vi "Variant to JSON Text.vi"(4 "LVClass Serializer":refnum<class "JSONtext LVClass Serializer.lvclass">, 5 "enable LabVIEW extensions? (T)":bool=TRUE, 6 "Pretty Print?":bool, 8 "error in (no error)":errorcluster, 10 "Variant":variant) -> (0 "error out":errorcluster, 1 "Name of data in Variant":string, 3 "<JSON>":string)   [LabVIEW 2017, in "JSONtext.lvlib"]
doc: "Converts a LabVIEW datatype (<b>Variant</b>) into a JSON value. \n\nStrings or Arrays of strings marked with a leading \"<JSON>\" tag in their name (including inside clusters) are treated as already being valid JSON. Strings not marked as <JSON> are quoted and escaped as a JSON String. Note that JSONtext.lvlib functions that produce JSON have their outputs labelled \"<JSON>\", so that they may be used as inputs to other functions.\n\nTwo types of LabVIEW Clusters are supported: either with all named elements, which are converted to JSON Objects, or all unnamed elements (or elements just named \"<JSON>\"), which are converted to a JSON Array. Handling of mixed clusters with some named and some unnamed in undefined (currently, this VI will use the first element to determine whether to convert to an Object or Array)."
uses:
  JSONtext.lvlib
  LVClass Serializer/JSONtext LVClass Serializer.lvclass
  <vilib>/Utility/Data Type/Type Definitions/Data Type.ctl
  support/Remove trailing zeros.vi
  support/quote and escape json string 2.vi
  support/Format JSON Object.vi
  <vilib>/Utility/Data Type/NI_Data Type.lvlib
  <vilib>/JDP Science/JDP Science Common Utilities/JDP Utility.lvlib
  <vilib>/JDP Science/JDP Science Common Utilities/Timestamp/JDP Timestamp.lvlib
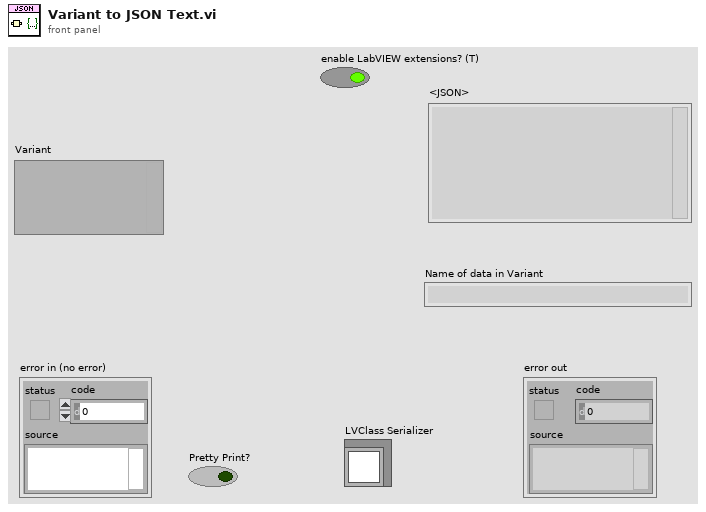
[diagram p1: front panel]
types:
  T1 = typedef "NI_Data Type.lvlib/Data Type.ctl" = enum8{"Invalid Type", "Void", "I8", "I16", "I32", "I64", "U8", "U16", "U32", "U64", "Single Float", "Double Float", "Extended Float", "Single Complex", "Double Complex", "Extended Complex", "Enum U8", "Enum U16", "Enum U32", "Enum U64", "Single Float With Unit", "Double Float With Unit", "Extended Float With Unit", "Single Complex with Unit", "Double Complex with Unit", "Extended Complex with Unit", "Boolean", "String", "Path", "Picture", "Tag", "Array", "Cluster", "Variant", "LV Variant", "Waveform", "Timestamp", "Digital Waveform", "Digital Data", "ExpressData", "Refnum", "External Data", "VI", "Poly VI", "LabVIEW Class Instance", "Fixed Point"}
  T2 = typedef "JSONtext.lvlib/Tag Type.ctl" = enum16{"No Tag", "<JSON>", "<JOBJ>"}
  T3 = cluster{"<JSON>attributes":string, "t0":timestamp, "dt":dbl, "Y":dbl[]}
  T4 = typedef "NI_Data Type.lvlib/Refnum Type.ctl" = enum16{"NotARefnum", "UnknownRefnum", "Generic", "Datalog", "ByteStream", "Device", "Occurence", "TCPNetConnection", "Auto", "Menu", "Imaq", "Hardware", "DataSocket", "Visa", "IVI", "UDPNetConnection", "Notifier", "Queue", "Irda", "EventReg", "DotNet", "UserEvent", "Callback", "UNUSED_EMPTY_POSITION", "BlueToothNetConnection", "LVObjApp", "LVObjVI", "LVObjUnknown", "GenericClass", "UserDefinedRefnumTag", "DataValue", "RT FIFO", "TDMS File"}
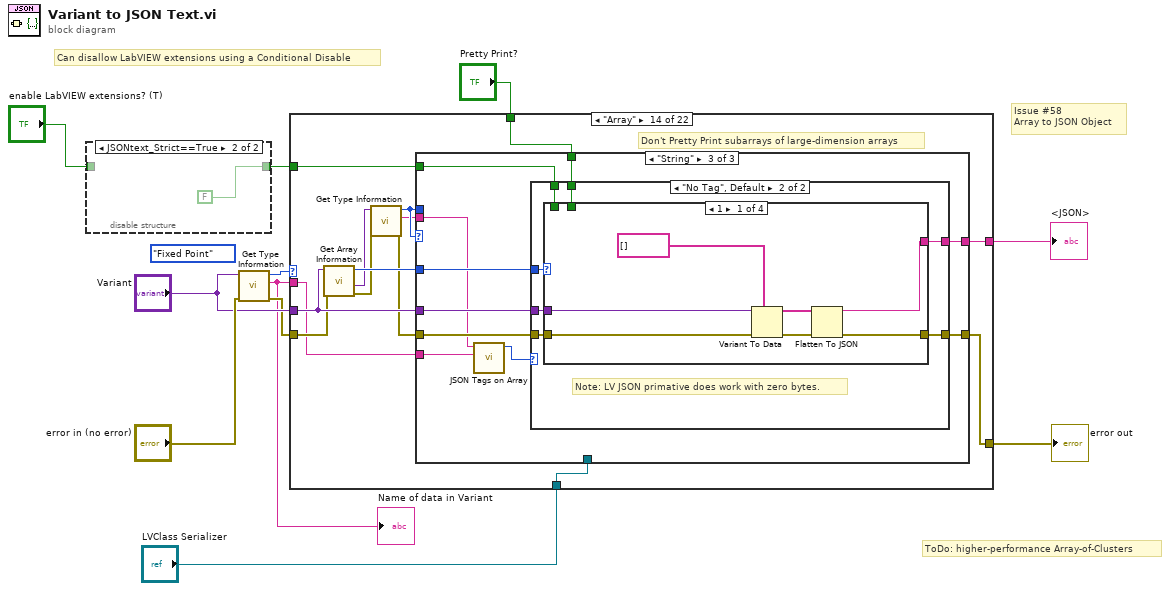
[diagram p0: block diagram]
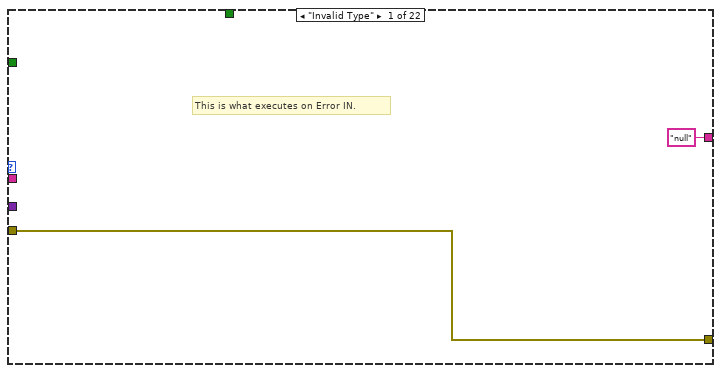
[diagram p3: hidden frame]
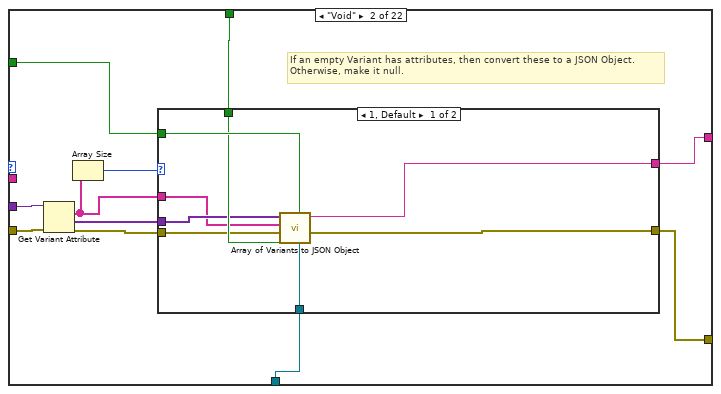
[diagram p4: hidden frame]
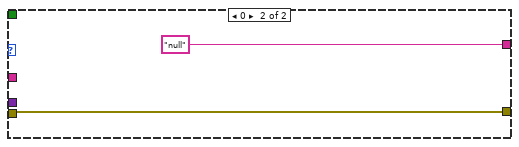
[diagram p5: hidden frame]
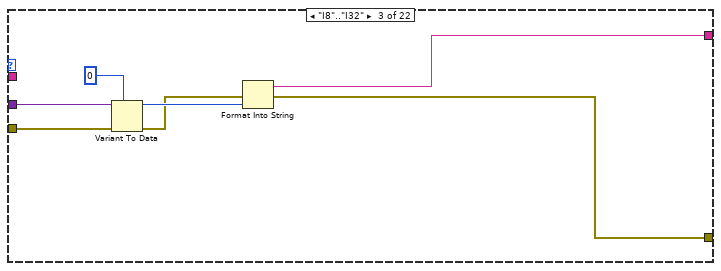
[diagram p6: hidden frame]
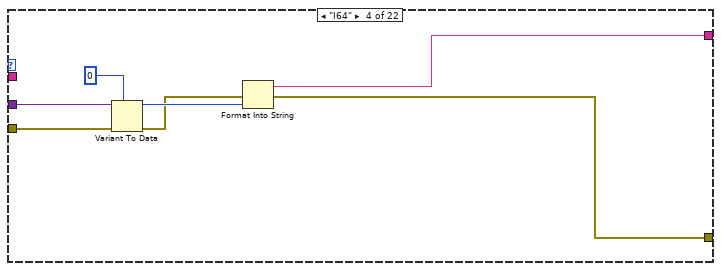
[diagram p7: hidden frame]
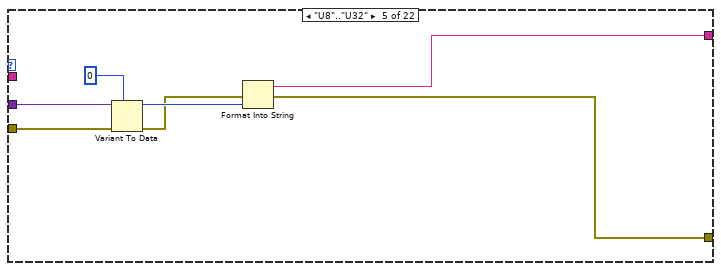
[diagram p8: hidden frame]
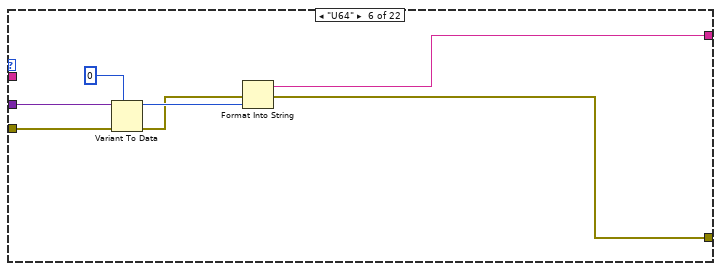
[diagram p9: hidden frame]
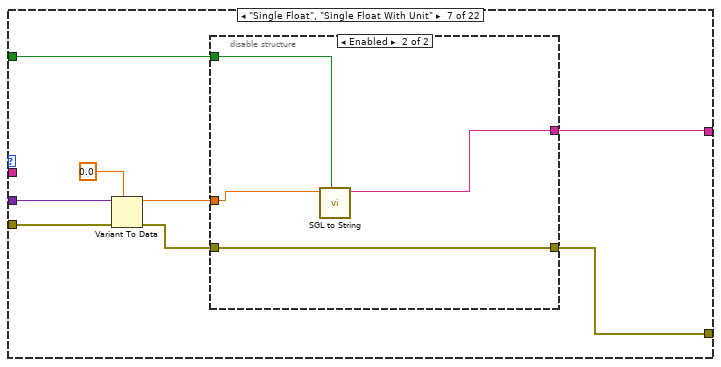
[diagram p10: hidden frame]
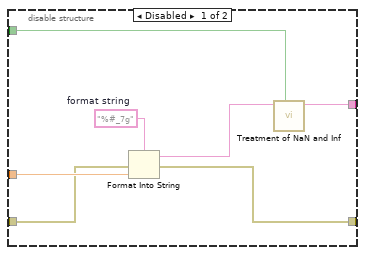
[diagram p11: hidden frame]
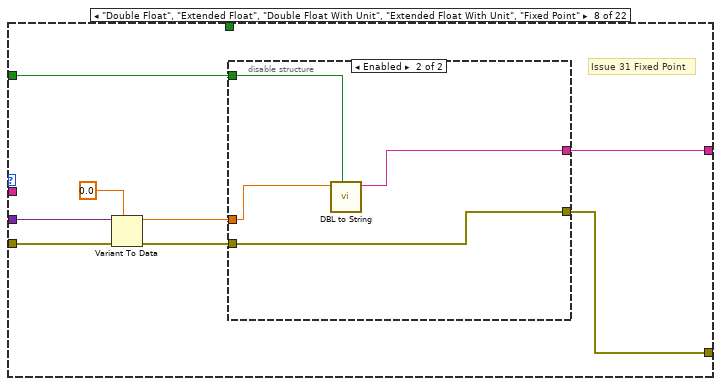
[diagram p12: hidden frame]
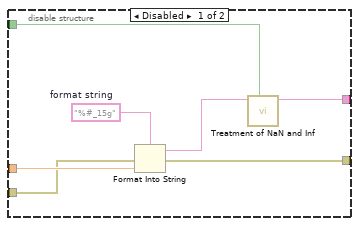
[diagram p13: hidden frame]
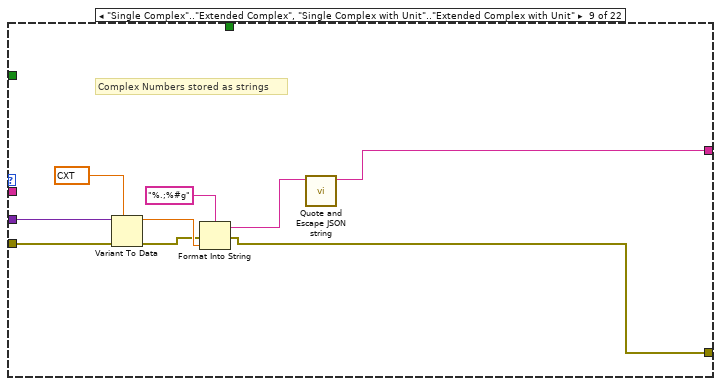
[diagram p14: hidden frame]
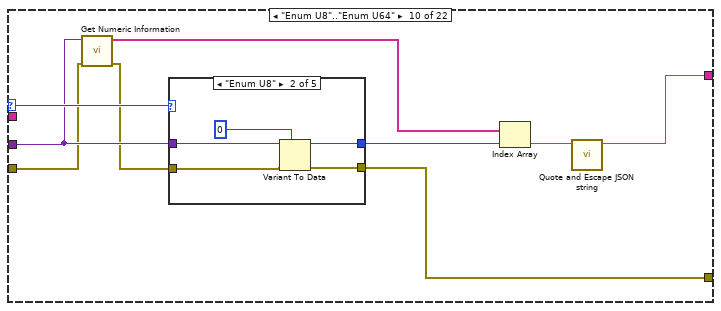
[diagram p15: hidden frame]
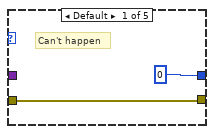
[diagram p16: hidden frame]
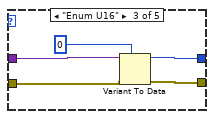
[diagram p17: hidden frame]
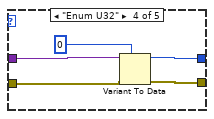
[diagram p18: hidden frame]
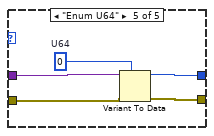
[diagram p19: hidden frame]
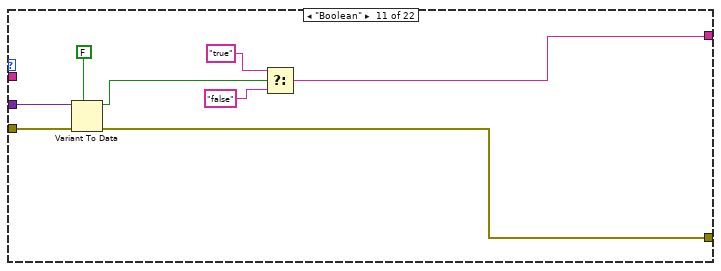
[diagram p20: hidden frame]
diagram:
  (unwired) Data_Type."Fixed Point" ("Type")
  # "ToDo: higher-performance Array-of-Clusters"
  # "Issue #58\nArray to JSON Object"
  # "Can disallow LabVIEW extensions using a Conditional Disable"
  n1 = disable-structure shown="JSONtext_Strict==True" {
    disable-tunnel: "enable LabVIEW extensions? (T)" -> [w12 _]
    disable-tunnel: [w12 FALSE ("enable LabVIEW extensions? (T)")] -> w3
    frame condition #0 (active) {
    }
    frame condition #1 {
    }
  }
  n2 = call <vilib>:"Get Type Information.vi"("error in (no error)"="error in (no error)", "Variant"="Variant") -> ("error out"=w6:errorcluster, "Name"=w4:string, "Type"=w5:T1)  [unwired: 5 in, 2 out]
  "Name of data in Variant" <- w4
  n3 = case shown="\"Array\"" w5 {
    selector: w5 -> [_ _ _ _ _ _ _ _ _ w119 _ _ _ _ _ _ _ _ _ _ _ _]
    tunnel: "Variant" -> [_ w25 w43 w50 w57 w64 w72 w91 w111 w115 w150 w159 w171 w184 w680 w700 w721 w756 w761 w785 w795 w809]
    tunnel: [w14 w26 w37 w44 w51 w58 w67 w86 w103 w114 w143 w155 w165 w185 w675 w704 w708 w750 w759 w783 w789 w806] -> w10
    tunnel: w6 -> [w14 w20 w41 w48 w55 w62 w70 w89 w110 w113 w148 w154 w169 w183 w678 w699 w720 w754 w760 w784 w794 w806]
    tunnel: w4 -> [_ _ _ _ _ _ _ _ _ _ _ w152 _ w175 _ _ _ _ _ _ _ _]
    tunnel: ["null" ("<JSON>") w19 w39 w46 w53 w60 w66 w85 w104 w117 w144 w153 w166 w177 w676 w696 w710 w751 w758 w782 w791 w807] -> w8
    tunnel: "Pretty Print?" -> [_ w18 _ _ _ _ _ _ _ _ _ _ _ w178 w674 w698 w707 _ _ _ _ _]
    tunnel: w3 -> [_ w17 _ _ _ _ w65 w84 _ _ _ _ _ w176 w670 w697 w706 _ _ _ _ _]
    tunnel: "LVClass Serializer" -> [_ w16 _ _ _ _ _ _ _ _ _ _ _ w172 w669 w695 w705 _ _ _ w786 _]
    frame "Invalid Type" {
      # "This is what executes on Error IN."
    }
    frame "Void" {
      # "If an empty Variant has attributes, then convert these to a JSON Object.\nOtherwise, make it null."
      n4 = Get Variant Attribute(Variant=w25, error in=w20) -> (names=w23:string[], values=w22:variant[], error out=w21:errorcluster)  [unwired: 2 in, 1 out]
      n5 = Array Size(array=w23) -> (size(s)=w24:i32)
      n6 = case shown="1, Default" w24 {
        tunnel: [w28 w35] -> w26
        tunnel: w23 -> [w30 _]
        tunnel: w22 -> [w31 _]
        tunnel: w21 -> [w29 w35]
        tunnel: [w34 "null"] -> w19
        tunnel: w18 -> [w32 _]
        tunnel: w17 -> [w33 _]
        tunnel: w16 -> [w27 _]
        frame 1, Default {
          n7 = call "Array of Variants to JSON Object.vi"("LVClass Serializer"=w27, "enable LabVIEW extensions? (T)"=w33, "Pretty Print?"=w32, "error in (no error)"=w29, "Names"=w30, "Array"=w31) -> ("error out"=w28:errorcluster, "<JSON>"=w34:string)  [unwired: 4 in]
        }
        frame 0 {
        }
      }
    }
    frame "I8".."I32" {
      n8 = Variant To Data(error in=w41, type=0, Variant=w43) -> (data=w40:i32, error out=w38:errorcluster)
      n9 = Format Into String(error in=w38, w40) -> (resulting string=w39:string, error out=w37:errorcluster)  [unwired: 2 in]
    }
    frame "I64" {
      n10 = Variant To Data(error in=w48, type=i64 0, Variant=w50) -> (data=w47:i64, error out=w45:errorcluster)
      n11 = Format Into String(error in=w45, w47) -> (resulting string=w46:string, error out=w44:errorcluster)  [unwired: 2 in]
    }
    frame "U8".."U32" {
      n12 = Variant To Data(error in=w55, type=u32 0, Variant=w57) -> (data=w54:u32, error out=w52:errorcluster)
      n13 = Format Into String(error in=w52, w54) -> (resulting string=w53:string, error out=w51:errorcluster)  [unwired: 2 in]
    }
    frame "U64" {
      n14 = Variant To Data(error in=w62, type=u64 0, Variant=w64) -> (data=w61:u64, error out=w59:errorcluster)
      n15 = Format Into String(error in=w59, w61) -> (resulting string=w60:string, error out=w58:errorcluster)  [unwired: 2 in]
    }
    frame "Single Float", "Single Float With Unit" {
      n16 = Variant To Data(error in=w70, type=sgl 0.0, Variant=w72) -> (data=w69:sgl, error out=w68:errorcluster)
      n17 = disable-structure shown="Enabled" {
        disable-tunnel: w69 -> [w79 w83]
        disable-tunnel: w68 -> [w78 w81]
        disable-tunnel: [w77 w81] -> w67
        disable-tunnel: [w74 w80] -> w66
        disable-tunnel: w65 -> [w73 w82]
        frame Disabled {
          w76 = "%#_7g"  # format string
          n18 = Format Into String(format string=w76, error in=w78, w79) -> (resulting string=w75:string, error out=w77:errorcluster)  [unwired: 1 in]
          n19 = call "Treatment of NaN and Inf.vi"("enable LabVIEW extensions?"=w73, "Numeric Text"=w75) -> ("<JSON>"=w74:string)  [unwired: 9 in]
        }
        frame Enabled {
          n20 = call "SGL to String.vi"("enable LabVIEW extensions?"=w82, "SGL"=w83) -> ("SGL string"=w80:string)  [unwired: 9 in]
        }
      }
    }
    frame "Double Float", "Extended Float", "Double Float With Unit", "Extended Float With Unit", "Fixed Point" {
      # "Issue 31 Fixed Point"
      n21 = Variant To Data(error in=w89, type=0.0, Variant=w91) -> (data=w88:dbl, error out=w87:errorcluster)
      n22 = disable-structure shown="Enabled" {
        disable-tunnel: w88 -> [w98 w102]
        disable-tunnel: w87 -> [w97 w99]
        disable-tunnel: [w96 w99] -> w86
        disable-tunnel: [w93 w101] -> w85
        disable-tunnel: w84 -> [w92 w100]
        frame Disabled {
          w95 = "%#_15g"  # format string
          n23 = Format Into String(format string=w95, error in=w97, w98) -> (resulting string=w94:string, error out=w96:errorcluster)  [unwired: 1 in]
          n24 = call "Treatment of NaN and Inf.vi"("enable LabVIEW extensions?"=w92, "Numeric Text"=w94) -> ("<JSON>"=w93:string)  [unwired: 9 in]
        }
        frame Enabled {
          n25 = call "DBL to String.vi"("enable LabVIEW extensions?"=w100, "DBL"=w102) -> ("DBL string"=w101:string)  [unwired: 9 in]
        }
      }
    }
    frame "Single Complex".."Extended Complex", "Single Complex with Unit".."Extended Complex with Unit" {
      # "Complex Numbers stored as strings"
      n26 = Variant To Data(error in=w110, type=cxt 0.0+0.0i, Variant=w111) -> (data=w108:cxt, error out=w107:errorcluster)
      n27 = Format Into String(format string="%.;%#g", error in=w107, w108) -> (resulting string=w105:string, error out=w103:errorcluster)  [unwired: 1 in]
      n28 = call "Quote and Escape JSON string.vi"("Plain Text"=w105) -> ("<JSON>"=w104:string)  [unwired: 10 in]
    }
    frame "Enum U8".."Enum U64" {
      n29 = call <vilib>:"Get Numeric Information.vi"("error in (no error)"=w113, "Variant"=w115) -> ("error out"=w112:errorcluster, "Enum Names"=w116:string[])  [unwired: 6 in, 2 out]
      n30 = case shown="\"Enum U8\"" w119 {
        tunnel: [u64 0 ("U8") w126 w131 w136 w141] -> w120
        tunnel: w115 -> [_ w125 w130 w135 w140]
        tunnel: w112 -> [w121 w124 w129 w134 w139]
        tunnel: [w121 w123 w128 w133 w138] -> w114
        frame Default {
          # "Can't happen"
        }
        frame "Enum U8" {
          n31 = Variant To Data(error in=w124, type=u8 0, Variant=w125) -> (data=w126:u8, error out=w123:errorcluster)
        }
        frame "Enum U16" {
          n32 = Variant To Data(error in=w129, type=u16 0, Variant=w130) -> (data=w131:u16, error out=w128:errorcluster)
        }
        frame "Enum U32" {
          n33 = Variant To Data(error in=w134, type=u32 0, Variant=w135) -> (data=w136:u32, error out=w133:errorcluster)
        }
        frame "Enum U64" {
          w142 = u64 0  # U64
          n34 = Variant To Data(error in=w139, type=w142, Variant=w140) -> (data=w141:u64, error out=w138:errorcluster)
        }
      }
      n35 = Index Array(array=w116, index=w120) -> (element=w118:string)
      n36 = call "Quote and Escape JSON string.vi"("Plain Text"=w118) -> ("<JSON>"=w117:string)  [unwired: 10 in]
    }
    frame "Boolean" {
      n37 = Variant To Data(error in=w148, type=FALSE, Variant=w150) -> (data=w145:bool, error out=w143:errorcluster)
      n38 = Select(t="true", s=w145, f="false") -> (s? t:f=w144:string)
    }
    frame "String" {
      n39 = Variant To Data(error in=w154, type="", Variant=w159) -> (data=w157:string, error out=w156:errorcluster)
      n40 = call "Remove JSON Tag.vi"("Name"=w152) -> ("Tag"=w151:T2)  [unwired: 9 in, 1 out]
      n41 = case shown="\"No Tag\", Default" w151 {
        tunnel: w157 -> [w162 w163]
        tunnel: w156 -> [w160 w164]
        tunnel: [w160 w164] -> w155
        tunnel: [w161 w163] -> w153
        frame "No Tag", Default {
          n42 = call "Quote and Escape JSON string.vi"("Plain Text"=w162) -> ("<JSON>"=w161:string)  [unwired: 10 in]
        }
        frame "<JSON>" {
          # "Already JSON"
        }
      }
    }
    frame "Path" {
      n43 = Variant To Data(error in=w169, type=path "", Variant=w171) -> (data=w168:path, error out=w165:errorcluster)
      n44 = Path To String(path=w168) -> (string=w167:string)
      n45 = call "Quote and Escape JSON string.vi"("Plain Text"=w167) -> ("<JSON>"=w166:string)  [unwired: 10 in]
    }
    frame "Array" {
      # "Don't Pretty Print subarrays of large-dimension arrays"
      n46 = call <vilib>:"Get Array Information.vi"("error in (no error)"=w183, "Variant"=w184) -> ("error out"=w181:errorcluster, "Array Element Data Type"=w180:variant, "Number of Dimensions"=w182:i32)  [unwired: 6 in, 1 out]
      n47 = call <vilib>:"Get Type Information.vi"("error in (no error)"=w181, "Variant"=w180) -> ("error out"=w179:errorcluster, "Name"=w173:string, "Type"=w174:T1)  [unwired: 5 in, 2 out]
      n48 = case shown="\"String\"" w174 {
        tunnel: [w186 w197 w597] -> w185
        tunnel: w184 -> [_ w196 w596]
        tunnel: w182 -> [_ w195 w595]
        tunnel: w179 -> [w186 w194 w594]
        tunnel: w174 -> [_ w193 _]
        tunnel: w178 -> [_ w192 w593]
        tunnel: ["null" ("JSON Object Text out") w191 w592] -> w177
        tunnel: w176 -> [_ w190 w591]
        tunnel: w175 -> [_ w189 w589]
        tunnel: w173 -> [_ _ w590]
        tunnel: w172 -> [_ w188 _]
        frame "Invalid Type" {
        }
        frame Default {
          n49 = case shown="1" w195 {
            selector: w195 -> [_ _ _ _ _ w581]
            tunnel: [w205 w359 w462 w555 w572 w587] -> w197
            tunnel: w196 -> [w206 w360 w463 w557 w574 _]
            tunnel: w194 -> [w204 w358 w461 w556 w573 w586]
            tunnel: w193 -> [w203 w357 w460 _ _ _]
            tunnel: w192 -> [w202 w356 w459 w548 w565 _]
            tunnel: [w201 w355 w458 w554 w571 "null" ("JSON Object Text out")] -> w191
            tunnel: w190 -> [w200 w354 w457 w549 w570 _]
            tunnel: w189 -> [w199 _ _ _ _ _]
            tunnel: w188 -> [w198 w353 w456 w547 w564 _]
            frame 1 {
              n50 = case shown="Default" w203 {
                tunnel: w206 -> [w214 w239 w256 w263 w284 w291 w298 w308 w321]
                tunnel: [w209 w234 w251 w258 w279 w286 w293 w301 w314] -> w205
                tunnel: w204 -> [w212 w237 w254 w261 w282 w289 w296 w306 w319]
                tunnel: w202 -> [_ _ _ _ _ _ _ w303 w316]
                tunnel: [w208 w233 w250 w257 w278 w285 w292 w304 w317] -> w201
                tunnel: w200 -> [w207 w232 _ _ _ _ _ w305 w318]
                tunnel: w199 -> [_ _ _ _ _ _ _ _ w312]
                tunnel: w198 -> [_ _ _ _ _ _ _ w299 w309]
                frame "Single Float" {
                  n51 = Variant To Data(error in=w212, type=sgl[] [], Variant=w214) -> (data=w211:sgl[], error out=w210:errorcluster)
                  n52 = disable-structure shown="Enabled" {
                    disable-tunnel: w211 -> [w219 w222 w228]
                    disable-tunnel: w210 -> [w218 w220 w230]
                    disable-tunnel: [w217 w220 w230] -> w209
                    disable-tunnel: [w216 w221 w231] -> w208
                    disable-tunnel: w207 -> [w215 _ w229]
                    frame Disabled {
                      # "Bug in 2015: Flatten to Json uses\n18 significant figures for SGL\ndata (reported to NI)."
                      n53 = Flatten To JSON(enable LabVIEW extensions? (T)=w215, anything=w219, error in (no error)=w218) -> (JSON string=w216:string, 11:w217:errorcluster)
                    }
                    frame Disabled {
                      w227 = "%_7g"  # format string
                      # "Not fast"
                      n54 = Array To Spreadsheet String(delimiter (Tab)=",", array=w222, 3:w227) -> (spreadsheet string=w225:string)
                      n55 = Concatenate Strings("[" ("string"), w225, "]" ("string")) -> (w221:string)
                    }
                    frame Enabled {
                      n56 = call "SGL Aray to JSON.vi"("enable LabVIEW extensions?"=w229, "SGL Array"=w228) -> ("<JSON>Array"=w231:string)  [unwired: 9 in]
                    }
                  }
                }
                frame "Double Float", "Extended Float" {
                  # "Bug in 2015: Flatten to Json uses\nonly 8 significant figures for EXT\ndata (reported to NI), so we \nconvert to DBLs"
                  n57 = Variant To Data(error in=w237, type=dbl[] [], Variant=w239) -> (data=w236:dbl[], error out=w235:errorcluster)
                  n58 = disable-structure shown="Enabled" {
                    disable-tunnel: w236 -> [w244 w248]
                    disable-tunnel: w235 -> [w243 w245]
                    disable-tunnel: [w242 w245] -> w234
                    disable-tunnel: [w241 w247] -> w233
                    disable-tunnel: w232 -> [w240 w246]
                    frame Disabled {
                      n59 = Flatten To JSON(enable LabVIEW extensions? (T)=w240, anything=w244, error in (no error)=w243) -> (JSON string=w241:string, 11:w242:errorcluster)
                    }
                    frame Enabled {
                      n60 = call "DBL Aray to JSON.vi"("enable LabVIEW extensions?"=w246, "DBL Array"=w248) -> ("<JSON>Array"=w247:string)  [unwired: 9 in]
                    }
                  }
                }
                frame "Path" {
                  n61 = Variant To Data(error in=w254, type=path[] [], Variant=w256) -> (data=w253:path[], error out=w252:errorcluster)
                  n62 = Path To String(path=w253) -> (string=w249:string[])
                  n63 = Flatten To JSON(anything=w249, error in (no error)=w252) -> (JSON string=w250:string, 11:w251:errorcluster)  [unwired: 1 in]
                }
                frame "I8".."I32" {
                  n64 = Variant To Data(error in=w261, type=i32[] [], Variant=w263) -> (data=w260:i32[], error out=w259:errorcluster)
                  n65 = disable-structure shown="Enabled" {
                    disable-tunnel: w260 -> [w267 w277]
                    disable-tunnel: w259 -> [w266 w268]
                    disable-tunnel: [w265 w268] -> w258
                    disable-tunnel: [w264 w273] -> w257
                    frame Enabled {
                      n66 = Flatten To JSON(anything=w267, error in (no error)=w266) -> (JSON string=w264:string, 11:w265:errorcluster)  [unwired: 1 in]
                    }
                    frame Disabled {
                      n67 = Array To Spreadsheet String(delimiter (Tab)=",", array=w277, 3:"%d" ("format string")) -> (spreadsheet string=w271:string)
                      n68 = call <vilib>:"Trim Whitespace__JDP.vi"("Remove (leading and trailing)"=enum16{"leading", "trailing", "both"}."trailing", "String in"=w271) -> ("String out"=w270:string)  [unwired: 5 in]
                      n69 = Concatenate Strings("[" ("string"), w270, "]" ("string")) -> (w273:string)
                    }
                  }
                }
                frame "I64" {
                  n70 = Variant To Data(error in=w282, type=i64[] [], Variant=w284) -> (data=w281:i64[], error out=w280:errorcluster)
                  n71 = Flatten To JSON(anything=w281, error in (no error)=w280) -> (JSON string=w278:string, 11:w279:errorcluster)  [unwired: 1 in]
                }
                frame "U8".."U32" {
                  n72 = Variant To Data(error in=w289, type=u32[] [], Variant=w291) -> (data=w288:u32[], error out=w287:errorcluster)
                  n73 = Flatten To JSON(anything=w288, error in (no error)=w287) -> (JSON string=w285:string, 11:w286:errorcluster)  [unwired: 1 in]
                }
                frame "U64" {
                  n74 = Variant To Data(error in=w296, type=u64[] [], Variant=w298) -> (data=w295:u64[], error out=w294:errorcluster)
                  n75 = Flatten To JSON(anything=w295, error in (no error)=w294) -> (JSON string=w292:string, 11:w293:errorcluster)  [unwired: 1 in]
                }
                frame Default {
                  # "Enums, etc."
                  n76 = Variant To Data(error in=w306, type=variant[] [], Variant=w308) -> (data=w300:variant[], error out=w302:errorcluster)
                  n77 = call "Array of Variants to JSON Array.vi"("LVClass Serializer"=w299, "enable LabVIEW extensions? (T)"=w305, "Pretty Print?"=w303, "error in (no error)"=w302, "Array of Variants"=w300) -> ("error out"=w301:errorcluster, "<JSON>"=w304:string)  [unwired: 5 in]
                }
                frame "Cluster" {
                  n78 = call "Remove OBJ Tag.vi"("Name"=w312) -> ("tagged as Item Name in JSON Objects"=w310:bool, "Name (tag stripped)"=w311:string)  [unwired: 9 in]
                  n79 = Variant To Data(error in=w319, type=variant[] [], Variant=w321) -> (data=w313:variant[], error out=w315:errorcluster)
                  n80 = case shown="True" w310 {
                    tunnel: w318 -> [w328 _]
                    tunnel: [w327 w331] -> w317
                    tunnel: w316 -> [w326 w330]
                    tunnel: w315 -> [w325 w336]
                    tunnel: [w324 w332] -> w314
                    tunnel: w313 -> [w323 w337]
                    tunnel: w311 -> [_ _]
                    tunnel: w309 -> [w322 w329]
                    frame False {
                      n81 = call "Array of Variants to JSON Array.vi"("LVClass Serializer"=w322, "enable LabVIEW extensions? (T)"=w328, "Pretty Print?"=w326, "error in (no error)"=w325, "Array of Variants"=w323) -> ("error out"=w324:errorcluster, "<JSON>"=w327:string)  [unwired: 5 in]
                    }
                    frame True {
                      n82 = for {
                        tunnel: w337 -> [w344] mode=indexing
                        shift-right: [w342] -> w333
                        shift-left: w336 -> [w347]
                        tunnel: [w341] -> w334 mode=indexing
                        tunnel: [w340] -> w335 mode=indexing
                        tunnel: w330 -> [w339]
                        tunnel: w329 -> [w338]
                        # "Issue #58 Cluster 1D Array to JOBJ"
                        n83 = Variant To Data(error in=w347, type=variant[] [], Variant=w344) -> (data=w343:variant[], error out=w346:errorcluster)
                        n84 = Index Array(array=w343) -> (element=w350:variant)  [unwired: 1 in]
                        n85 = Array Subset(array=w343, index=1) -> (w351:variant[])  [unwired: 1 in]
                        n86 = Variant To Data(error in=w346, type="", Variant=w350) -> (data=w340:string, error out=w349:errorcluster)
                        n87 = call "Array of Variants to JSON Object.vi"("LVClass Serializer"=w338, "Pretty Print?"=w339, "error in (no error)"=w349, "Array"=w351) -> ("error out"=w342:errorcluster, "<JSON>"=w341:string)  [unwired: 6 in]
                      }
                      n88 = call "Make JSON Object.vi"("Pretty Print?"=w330, "error in (no error)"=w333, "JSON Items"=w334, "Item Names"=w335) -> ("error out"=w332:errorcluster, "<JSON>"=w331:string)  [unwired: 6 in]
                    }
                  }
                }
              }
            }
            frame 2 {
              n89 = case shown="Default" w357 {
                tunnel: w360 -> [w369 w393 w415 w422 w429 w436 w448]
                tunnel: [w364 w388 w410 w417 w424 w431 w440] -> w359
                tunnel: w358 -> [w367 w391 w413 w420 w427 w434 w446]
                tunnel: w356 -> [w361 w385 _ _ _ _ w438]
                tunnel: [w363 w387 w409 w416 w423 w430 w439] -> w355
                tunnel: w354 -> [w362 w386 _ _ _ _ w443]
                tunnel: w353 -> [_ _ _ _ _ _ w437]
                frame "Single Float" {
                  n90 = Variant To Data(error in=w367, type=sgl[][] [], Variant=w369) -> (data=w366:sgl[][], error out=w365:errorcluster)
                  n91 = disable-structure shown="Enabled" {
                    disable-tunnel: w366 -> [w374 w381]
                    disable-tunnel: w365 -> [w373 w377]
                    disable-tunnel: [w372 w378] -> w364
                    disable-tunnel: [w371 w379] -> w363
                    disable-tunnel: w362 -> [w370 w376]
                    disable-tunnel: w361 -> [_ w375]
                    frame Disabled {
                      # "Bug in 2015: Flatten to Json uses\n18 significant figures for SGL\ndata (reported to NI)."
                      n92 = Flatten To JSON(enable LabVIEW extensions? (T)=w370, anything=w374, error in (no error)=w373) -> (JSON string=w371:string, 11:w372:errorcluster)
                    }
                    frame Enabled {
                      n93 = for {
                        tunnel: w381 -> [w384] mode=indexing
                        tunnel: [w383] -> w380 mode=indexing
                        tunnel: w376 -> [w382]
                        n94 = call "SGL Aray to JSON.vi"("enable LabVIEW extensions?"=w382, "SGL Array"=w384) -> ("<JSON>Array"=w383:string)  [unwired: 9 in]
                      }
                      n95 = call "Format JSON Array Text.vi"("Pretty Print?"=w375, "error in (no error)"=w377, "Array of JSON Text"=w380) -> ("error out"=w378:errorcluster, "<JSON>"=w379:string)  [unwired: 7 in]
                    }
                  }
                }
                frame "Double Float", "Extended Float" {
                  # "No easy way to support full EXT precision"
                  n96 = Variant To Data(error in=w391, type=dbl[][] [], Variant=w393) -> (data=w390:dbl[][], error out=w389:errorcluster)
                  n97 = disable-structure shown="Enabled" {
                    disable-tunnel: w390 -> [w398 w404]
                    disable-tunnel: w389 -> [w397 w403]
                    disable-tunnel: [w396 w402] -> w388
                    disable-tunnel: [w395 w401] -> w387
                    disable-tunnel: w386 -> [w394 w400]
                    disable-tunnel: w385 -> [_ w399]
                    frame Disabled {
                      # "Bug in 2015: Flatten to Json uses\n9 significant figures for EXT\ndata (reported to NI)."
                      n98 = Flatten To JSON(enable LabVIEW extensions? (T)=w394, anything=w398, error in (no error)=w397) -> (JSON string=w395:string, 11:w396:errorcluster)
                    }
                    frame Enabled {
                      n99 = for {
                        tunnel: w404 -> [w408] mode=indexing
                        tunnel: [w407] -> w405 mode=indexing
                        tunnel: w400 -> [w406]
                        n100 = call "DBL Aray to JSON.vi"("enable LabVIEW extensions?"=w406, "DBL Array"=w408) -> ("<JSON>Array"=w407:string)  [unwired: 9 in]
                      }
                      n101 = call "Format JSON Array Text.vi"("Pretty Print?"=w399, "error in (no error)"=w403, "Array of JSON Text"=w405) -> ("error out"=w402:errorcluster, "<JSON>"=w401:string)  [unwired: 7 in]
                    }
                  }
                }
                frame "I8".."I32" {
                  n102 = Variant To Data(error in=w413, type=i32[][] [], Variant=w415) -> (data=w412:i32[][], error out=w411:errorcluster)
                  n103 = Flatten To JSON(anything=w412, error in (no error)=w411) -> (JSON string=w409:string, 11:w410:errorcluster)  [unwired: 1 in]
                }
                frame "I64" {
                  n104 = Variant To Data(error in=w420, type=i64[][] [], Variant=w422) -> (data=w419:i64[][], error out=w418:errorcluster)
                  n105 = Flatten To JSON(anything=w419, error in (no error)=w418) -> (JSON string=w416:string, 11:w417:errorcluster)  [unwired: 1 in]
                }
                frame "U8".."U32" {
                  n106 = Variant To Data(error in=w427, type=u32[][] [], Variant=w429) -> (data=w426:u32[][], error out=w425:errorcluster)
                  n107 = Flatten To JSON(anything=w426, error in (no error)=w425) -> (JSON string=w423:string, 11:w424:errorcluster)  [unwired: 1 in]
                }
                frame "U64" {
                  n108 = Variant To Data(error in=w434, type=u64[][] [], Variant=w436) -> (data=w433:u64[][], error out=w432:errorcluster)
                  n109 = Flatten To JSON(anything=w433, error in (no error)=w432) -> (JSON string=w430:string, 11:w431:errorcluster)  [unwired: 1 in]
                }
                frame Default {
                  n110 = Variant To Data(error in=w446, type=variant[][] [], Variant=w448) -> (data=w441:variant[][], error out=w442:errorcluster)
                  n111 = for {
                    tunnel: w441 -> [w455] mode=indexing
                    tunnel: [w451] -> w444 mode=indexing
                    shift-right: [w454] -> w445
                    shift-left: w442 -> [w453]
                    tunnel: w443 -> [w452]
                    tunnel: w437 -> [w449]
                    n112 = call "Variant to JSON Text.vi"("LVClass Serializer"=w449, "enable LabVIEW extensions? (T)"=w452, "Pretty Print?"=FALSE, "error in (no error)"=w453, "Variant"=w455) -> ("error out"=w454:errorcluster, "<JSON>"=w451:string)  [unwired: 4 in, 1 out]
                  }
                  n113 = call "Format JSON Array Text.vi"("Pretty Print?"=w438, "error in (no error)"=w445, "Array of JSON Text"=w444) -> ("error out"=w440:errorcluster, "<JSON>"=w439:string)  [unwired: 7 in]
                }
              }
            }
            frame 3 {
              n114 = case shown="Default" w460 {
                tunnel: w463 -> [w475 w493 w507 w514 w521 w528 w540]
                tunnel: [w470 w489 w502 w509 w516 w523 w532] -> w462
                tunnel: w461 -> [w473 w491 w505 w512 w519 w526 w538]
                tunnel: w459 -> [w465 w483 _ _ _ _ w530]
                tunnel: [w469 w488 w501 w508 w515 w522 w531] -> w458
                tunnel: w457 -> [w468 w487 w500 _ _ _ w535]
                tunnel: w456 -> [w464 w482 _ _ _ _ w529]
                frame "Single Float" {
                  n115 = Variant To Data(error in=w473, type=sgl[][][] [], Variant=w475) -> (data=w472:sgl[][][], error out=w471:errorcluster)
                  n116 = for {
                    tunnel: w472 -> [w481] mode=indexing
                    tunnel: [w479] -> w467 mode=indexing
                    tunnel: w468 -> [w480]
                    shift-right: [w477] -> w466
                    shift-left: w471 -> [w478]
                    tunnel: w464 -> [w476]
                    n117 = call "Variant to JSON Text.vi"("LVClass Serializer"=w476, "enable LabVIEW extensions? (T)"=w480, "error in (no error)"=w478, "Variant"=w481) -> ("error out"=w477:errorcluster, "<JSON>"=w479:string)  [unwired: 5 in, 1 out]
                  }
                  n118 = call "Format JSON Array Text.vi"("Pretty Print?"=w465, "error in (no error)"=w466, "Array of JSON Text"=w467) -> ("error out"=w470:errorcluster, "<JSON>"=w469:string)  [unwired: 7 in]
                }
                frame "Double Float", "Extended Float" {
                  n119 = Variant To Data(error in=w491, type=dbl[][][] [], Variant=w493) -> (data=w490:dbl[][][], error out=w485:errorcluster)
                  n120 = for {
                    tunnel: w490 -> [w498] mode=indexing
                    tunnel: [w497] -> w486 mode=indexing
                    tunnel: w487 -> [w499]
                    shift-right: [w495] -> w484
                    shift-left: w485 -> [w496]
                    tunnel: w482 -> [w494]
                    n121 = call "Variant to JSON Text.vi"("LVClass Serializer"=w494, "enable LabVIEW extensions? (T)"=w499, "error in (no error)"=w496, "Variant"=w498) -> ("error out"=w495:errorcluster, "<JSON>"=w497:string)  [unwired: 5 in, 1 out]
                  }
                  n122 = call "Format JSON Array Text.vi"("Pretty Print?"=w483, "error in (no error)"=w484, "Array of JSON Text"=w486) -> ("error out"=w489:errorcluster, "<JSON>"=w488:string)  [unwired: 7 in]
                }
                frame "I8".."I32" {
                  n123 = Variant To Data(error in=w505, type=i32[][][] [], Variant=w507) -> (data=w504:i32[][][], error out=w503:errorcluster)
                  n124 = Flatten To JSON(enable LabVIEW extensions? (T)=w500, anything=w504, error in (no error)=w503) -> (JSON string=w501:string, 11:w502:errorcluster)
                }
                frame "I64" {
                  n125 = Variant To Data(error in=w512, type=i64[][][] [], Variant=w514) -> (data=w511:i64[][][], error out=w510:errorcluster)
                  n126 = Flatten To JSON(anything=w511, error in (no error)=w510) -> (JSON string=w508:string, 11:w509:errorcluster)  [unwired: 1 in]
                }
                frame "U8".."U32" {
                  n127 = Variant To Data(error in=w519, type=u32[][][] [], Variant=w521) -> (data=w518:u32[][][], error out=w517:errorcluster)
                  n128 = Flatten To JSON(anything=w518, error in (no error)=w517) -> (JSON string=w515:string, 11:w516:errorcluster)  [unwired: 1 in]
                }
                frame "U64" {
                  n129 = Variant To Data(error in=w526, type=u64[][][] [], Variant=w528) -> (data=w525:u64[][][], error out=w524:errorcluster)
                  n130 = Flatten To JSON(anything=w525, error in (no error)=w524) -> (JSON string=w522:string, 11:w523:errorcluster)  [unwired: 1 in]
                }
                frame Default {
                  n131 = Variant To Data(error in=w538, type=variant[][][] [], Variant=w540) -> (data=w533:variant[][][], error out=w534:errorcluster)
                  n132 = for {
                    tunnel: w533 -> [w546] mode=indexing
                    tunnel: [w542] -> w536 mode=indexing
                    shift-right: [w545] -> w537
                    shift-left: w534 -> [w544]
                    tunnel: w535 -> [w543]
                    tunnel: w529 -> [w541]
                    n133 = call "Variant to JSON Text.vi"("LVClass Serializer"=w541, "enable LabVIEW extensions? (T)"=w543, "error in (no error)"=w544, "Variant"=w546) -> ("error out"=w545:errorcluster, "<JSON>"=w542:string)  [unwired: 5 in, 1 out]
                  }
                  n134 = call "Format JSON Array Text.vi"("Pretty Print?"=w530, "error in (no error)"=w537, "Array of JSON Text"=w536) -> ("error out"=w532:errorcluster, "<JSON>"=w531:string)  [unwired: 7 in]
                }
              }
            }
            frame 4 {
              n135 = Variant To Data(error in=w556, type=variant[][][][] [], Variant=w557) -> (data=w552:variant[][][][], error out=w551:errorcluster)
              n136 = for {
                tunnel: w552 -> [w563] mode=indexing
                shift-right: [w561] -> w555
                shift-left: w551 -> [w562]
                tunnel: [w559] -> w550 mode=indexing
                tunnel: w549 -> [w560]
                tunnel: w547 -> [w558]
                n137 = call "Variant to JSON Text.vi"("LVClass Serializer"=w558, "enable LabVIEW extensions? (T)"=w560, "error in (no error)"=w562, "Variant"=w563) -> ("error out"=w561:errorcluster, "<JSON>"=w559:string)  [unwired: 5 in, 1 out]
              }
              n138 = call "Format JSON Array Text.vi"("Pretty Print?"=w548, "Array of JSON Text"=w550) -> ("<JSON>"=w554:string)  [unwired: 8 in, 1 out]
            }
            frame 5 {
              n139 = Variant To Data(error in=w573, type=variant[][][][][] [], Variant=w574) -> (data=w568:variant[][][][][], error out=w567:errorcluster)
              n140 = for {
                tunnel: w568 -> [w580] mode=indexing
                shift-right: [w578] -> w572
                shift-left: w567 -> [w579]
                tunnel: [w576] -> w566 mode=indexing
                tunnel: w570 -> [w577]
                tunnel: w564 -> [w575]
                n141 = call "Variant to JSON Text.vi"("LVClass Serializer"=w575, "enable LabVIEW extensions? (T)"=w577, "error in (no error)"=w579, "Variant"=w580) -> ("error out"=w578:errorcluster, "<JSON>"=w576:string)  [unwired: 5 in, 1 out]
              }
              n142 = call "Format JSON Array Text.vi"("Pretty Print?"=w565, "Array of JSON Text"=w566) -> ("<JSON>"=w571:string)  [unwired: 8 in, 1 out]
            }
            frame Default {
              n143 = Format Into String(format string="Can't support array of dim=%d", w581) -> (resulting string=w584:string)  [unwired: 2 in, 1 out]
              n144 = call <vilib>:"Error Cluster From Error Code.vi"("error in (no error)"=w586, "error message (\"\")"=w584, "error code (0)"=402843) -> ("error out"=w587:errorcluster)  [unwired: 6 in]
            }
          }
        }
        frame "String" {
          n145 = call "JSON Tags on Array.vi"("Array Name"=w589, "Element Name"=w590) -> ("Tag"=w588:T2)  [unwired: 9 in]
          n146 = case shown="\"No Tag\", Default" w588 {
            tunnel: [w601 w640] -> w597
            tunnel: w596 -> [w604 w639]
            tunnel: w595 -> [w598 w638]
            tunnel: w594 -> [w603 w637]
            tunnel: w593 -> [w599 w636]
            tunnel: [w602 w635] -> w592
            tunnel: w591 -> [w600 w634]
            frame "<JSON>" {
              # "JSON text --> can't use LV primative"
              n147 = case shown="0, Default" w598 {
                selector: w598 -> [w606 _ _]
                tunnel: w604 -> [_ w618 w628]
                tunnel: w603 -> [w607 w617 w627]
                tunnel: ["null" ("<JSON>") w615 w620] -> w602
                tunnel: [w605 w616 w622] -> w601
                tunnel: w600 -> [_ _ _]
                tunnel: w599 -> [_ w614 w621]
                frame 0, Default {
                  n148 = Format Into String(format string="Can't support array of dim=%d", w606) -> (resulting string=w609:string)  [unwired: 2 in, 1 out]
                  n149 = call <vilib>:"Error Cluster From Error Code.vi"("error in (no error)"=w607, "error message (\"\")"=w609, "error code (0)"=402843) -> ("error out"=w605:errorcluster)  [unwired: 6 in]
                }
                frame 1 {
                  n150 = Variant To Data(error in=w617, type=string[] [], Variant=w618) -> (data=w612:string[], error out=w613:errorcluster)
                  n151 = call "Format JSON Array Text.vi"("Pretty Print?"=w614, "error in (no error)"=w613, "Array of JSON Text"=w612) -> ("error out"=w616:errorcluster, "<JSON>"=w615:string)  [unwired: 7 in]
                }
                frame 2 {
                  n152 = Variant To Data(error in=w627, type=string[][] [], Variant=w628) -> (data=w625:string[][], error out=w626:errorcluster)
                  n153 = for {
                    tunnel: [w632] -> w624 mode=indexing
                    tunnel: w625 -> [w630] mode=indexing
                    shift-right: [w633] -> w623
                    shift-left: w626 -> [w631]
                    n154 = call "Format JSON Array Text.vi"("error in (no error)"=w631, "Array of JSON Text"=w630) -> ("error out"=w633:errorcluster, "<JSON>"=w632:string)  [unwired: 8 in]
                  }
                  n155 = call "Format JSON Array Text.vi"("Pretty Print?"=w621, "error in (no error)"=w623, "Array of JSON Text"=w624) -> ("error out"=w622:errorcluster, "<JSON>"=w620:string)  [unwired: 7 in]
                }
              }
            }
            frame "No Tag", Default {
              # "Note: LV JSON primative does work with zero bytes."
              n156 = case shown="1" w638 {
                selector: w638 -> [_ _ _ w662]
                tunnel: [w646 w653 w660 w668] -> w640
                tunnel: w639 -> [w647 w654 w661 _]
                tunnel: w637 -> [w645 w652 w659 w667]
                tunnel: w636 -> [_ _ _ _]
                tunnel: [w644 w651 w658 "null" ("JSON Object Text out")] -> w635
                tunnel: w634 -> [_ _ _ _]
                frame 1 {
                  n157 = Variant To Data(error in=w645, type=string[] [], Variant=w647) -> (data=w642:string[], error out=w641:errorcluster)
                  n158 = Flatten To JSON(anything=w642, error in (no error)=w641) -> (JSON string=w644:string, 11:w646:errorcluster)  [unwired: 1 in]
                }
                frame 2 {
                  n159 = Variant To Data(error in=w652, type=string[][] [], Variant=w654) -> (data=w649:string[][], error out=w648:errorcluster)
                  n160 = Flatten To JSON(anything=w649, error in (no error)=w648) -> (JSON string=w651:string, 11:w653:errorcluster)  [unwired: 1 in]
                }
                frame 3 {
                  n161 = Variant To Data(error in=w659, type=string[][][] [], Variant=w661) -> (data=w656:string[][][], error out=w655:errorcluster)
                  n162 = Flatten To JSON(anything=w656, error in (no error)=w655) -> (JSON string=w658:string, 11:w660:errorcluster)  [unwired: 1 in]
                }
                frame Default {
                  n163 = Format Into String(format string="Can't support array of dim=%d", w662) -> (resulting string=w665:string)  [unwired: 2 in, 1 out]
                  n164 = call <vilib>:"Error Cluster From Error Code.vi"("error in (no error)"=w667, "error message (\"\")"=w665, "error code (0)"=402843) -> ("error out"=w668:errorcluster)  [unwired: 6 in]
                }
              }
            }
          }
        }
      }
    }
    frame "Cluster" {
      # "Cluster of unnamed (possibly with <JSON>tags) to JSON Array?"
      n165 = Variant To Data(error in=w678, type=variant[] [], Variant=w680) -> (data=w673:variant[], error out=w679:errorcluster)
      n166 = Index Array(array=w673) -> (element=w672:variant)  [unwired: 1 in]
      n167 = call <vilib>:"Get Type Information.vi"("Variant"=w672) -> ("Name"=w671:string)  [unwired: 6 in, 4 out]
      n168 = case shown="Default" w671 {
        tunnel: w679 -> [w684 w690]
        tunnel: [w682 w694] -> w676
        tunnel: [w683 w689] -> w675
        tunnel: w674 -> [w686 w692]
        tunnel: w673 -> [w685 w691]
        tunnel: w670 -> [w687 w693]
        tunnel: w669 -> [w681 w688]
        frame Default {
          n169 = call "Array of Variants to JSON Object.vi"("LVClass Serializer"=w681, "enable LabVIEW extensions? (T)"=w687, "Pretty Print?"=w686, "error in (no error)"=w684, "Array"=w685) -> ("error out"=w683:errorcluster, "<JSON>"=w682:string)  [unwired: 5 in]
        }
        frame "", "<JSON>" {
          n170 = call "Array of Variants to JSON Array.vi"("LVClass Serializer"=w688, "enable LabVIEW extensions? (T)"=w693, "Pretty Print?"=w692, "error in (no error)"=w690, "Array of Variants"=w691) -> ("error out"=w689:errorcluster, "<JSON>"=w694:string)  [unwired: 5 in]
        }
      }
    }
    frame "Variant", "LV Variant" {
      n171 = Variant To Data(error in=w699, type=variant, Variant=w700) -> (data=w703:variant, error out=w702:errorcluster)
      n172 = call "Variant to JSON Text.vi"("LVClass Serializer"=w695, "enable LabVIEW extensions? (T)"=w697, "Pretty Print?"=w698, "error in (no error)"=w702, "Variant"=w703) -> ("error out"=w704:errorcluster, "<JSON>"=w696:string)  [unwired: 4 in, 1 out]
    }
    frame "Waveform" {
      n173 = Variant To Data(error in=w720, type=waveform(dbl) {"t0"=timestamp(0 s since 1904-01-01), "dt"=1.0, "Y"=[]} ("waveform"), Variant=w721) -> (data=w718:waveform(dbl), error out=w709:errorcluster)
      n174 = Unbundle By Name(w718) -> ("t0"=w717:timestamp, "dt"=w716:dbl, "Y"=w715:dbl[], "attributes"=w714:variant)
      n175 = Get Variant Attribute(Variant=w714) -> (names=w711:string[], values=w712:variant[])  [unwired: 3 in, 2 out]
      n176 = Array Size(array=w711) -> (size(s)=w713:i32)
      n177 = case shown="0" w713 {
        tunnel: w717 -> [w731 w749]
        tunnel: w716 -> [w730 w748]
        tunnel: w715 -> [w729 w747]
        tunnel: [w723 w739] -> w710
        tunnel: w712 -> [_ w736]
        tunnel: w711 -> [_ w733]
        tunnel: w707 -> [w724 w738]
        tunnel: w709 -> [w727 w735]
        tunnel: [w726 w743] -> w708
        tunnel: w706 -> [w725 w740]
        tunnel: w706 -> [_ w737]
        tunnel: w705 -> [w722 w732]
        frame 0 {
          # "No Attributes"
          n178 = Bundle("t0"=w731, "dt"=w730, "Y"=w729) -> (w728:cluster{"t0":timestamp, "dt":dbl, "Y":dbl[]})  [unwired: 1 in]
          n179 = call "Variant to JSON Text.vi"("LVClass Serializer"=w722, "enable LabVIEW extensions? (T)"=w725, "Pretty Print?"=w724, "error in (no error)"=w727, "Variant"=w728) -> ("error out"=w726:errorcluster, "<JSON>"=w723:string)  [unwired: 4 in, 1 out]
        }
        frame Default {
          w745 = ""  # <JSON>attributes
          n180 = call "Array of Variants to JSON Object.vi"("LVClass Serializer"=w732, "enable LabVIEW extensions? (T)"=w737, "Pretty Print?"=w737, "error in (no error)"=w735, "Names"=w733, "Array"=w736) -> ("error out"=w734:errorcluster, "<JSON>"=w746:string)  [unwired: 4 in]
          n181 = Variant To Data(error in=w734, type=w745, Variant=w746) -> (data=w741:string, error out=w742:errorcluster)
          n182 = Bundle("<JSON>attributes"=w741, "t0"=w749, "dt"=w748, "Y"=w747) -> (w744:T3)  [unwired: 1 in]
          n183 = call "Variant to JSON Text.vi"("LVClass Serializer"=w732, "enable LabVIEW extensions? (T)"=w740, "Pretty Print?"=w738, "error in (no error)"=w742, "Variant"=w744) -> ("error out"=w743:errorcluster, "<JSON>"=w739:string)  [unwired: 4 in, 1 out]
        }
      }
    }
    frame "Timestamp" {
      n184 = Variant To Data(error in=w754, type=timestamp(0 s since 1904-01-01), Variant=w756) -> (data=w753:timestamp, error out=w750:errorcluster)
      n185 = call <vilib>:"Timestamp to Text.vi"("Time Stamp"=w753) -> ("Timestamp (RFC3339)"=w752:string)  [unwired: 9 in, 1 out]
      n186 = call "Quote and Escape JSON string.vi"("Plain Text"=w752) -> ("<JSON>"=w751:string)  [unwired: 10 in]
    }
    frame "Refnum" {
      n187 = call <vilib>:"Get Refnum Information.vi"("error in (no error)"=w760, "Variant"=w761) -> ("error out"=w763:errorcluster, "Reference Type"=w762:T4)  [unwired: 6 in, 2 out]
      n188 = case shown="Default" w762 {
        selector: w762 -> [_ _ w774]
        tunnel: ["null" w767 w775] -> w757
        tunnel: w763 -> [w764 w769 w777]
        tunnel: [w764 w766 w776] -> w759
        tunnel: w761 -> [_ w770 w779]
        frame "NotARefnum", "UnknownRefnum" {
        }
        frame "Visa", "IVI", "UserDefinedRefnumTag" {
          n189 = Variant To Data(error in=w769, type="", Variant=w770) -> (data=w767:string, error out=w766:errorcluster)
        }
        frame Default {
          # "Store refnums in Hex (use case: routing back replies)"
          n190 = Variant To Flattened String(Variant=w779) -> (data string=w778:string)  [unwired: 1 out]
          n191 = Type Cast(type=u32 0, x=w778) -> (*(type *) &x=w771:u32)
          n192 = Format Into String(format string="%s->%x", error in=w777, w774, w771) -> (resulting string=w775:string, error out=w776:errorcluster)  [unwired: 1 in]
        }
      }
      n193 = call "Quote and Escape JSON string.vi"("Plain Text"=w757) -> ("<JSON>"=w758:string)  [unwired: 10 in]
    }
    frame "Tag" {
      # "Issue 37, handle DAQmx Tags"
      n194 = Variant To Data(error in=w784, type="", Variant=w785) -> (data=w781:string, error out=w783:errorcluster)
      n195 = call "Quote and Escape JSON string.vi"("Plain Text"=w781) -> ("<JSON>"=w782:string)  [unwired: 10 in]
    }
    frame "LabVIEW Class Instance" {
      w788 = refnum<class "JSONtext LVClass Serializer.lvclass"> refnum  # Default Flattening
      n196 = Variant To Data(error in=w794, type=refnum<class> refnum ("LabVIEW Object"), Variant=w795) -> (data=w792:refnum<class>, error out=w790:errorcluster)
      n197 = Not Equal?(x=w786, y=w788) -> (x != y?=w787:bool)
      n198 = case shown="False" w787 {
        tunnel: w792 -> [w800 w802]
        tunnel: [w799 w803] -> w791
        tunnel: w790 -> [w797 w805]
        tunnel: [w796 w804] -> w789
        tunnel: w786 -> [_ w801]
        frame False {
          # "Default Flattening:\nClasses saved in flattened form as strings"
          n199 = Flatten To String(anything=w800, error in (no error)=w797) -> (data string=w798:string, error out=w796:errorcluster)  [unwired: 2 in, 1 out]
          n200 = call "Quote and Escape JSON string.vi"("Plain Text"=w798) -> ("<JSON>"=w799:string)  [unwired: 10 in]
        }
        frame True {
          # "Issue #56 Way of providing alternate format\nof LVObjects"
          n201 = call-dynamic "LVObject to JSON.vi"("JSONtext LVClass Serializer in"=w801, "error in (no error)"=w805, "Object"=w802) -> ("error out"=w804:errorcluster, "<JSON>Object"=w803:string)  [unwired: 7 in]
        }
      }
    }
    frame Default {
      # "For lack of a better thing to do,\nflatten to string."
      n202 = Variant To Flattened String(Variant=w809) -> (data string=w808:string)  [unwired: 1 out]
      n203 = call "Quote and Escape JSON string.vi"("Plain Text"=w808) -> ("<JSON>"=w807:string)  [unwired: 10 in]
    }
  }
  "error out" <- w10
  "<JSON>" <- w8
